vi "Serial_numberExt_429B.vi"(10 "PCBA Barcode":string="SVI77664916000894", 11 "Test Operator ID":string="13984") -> (0 "Check SUM HEX":string, 1 "Serial number (Hex)":string, 3 "ProgrammingResult":bool)   [LabVIEW 2018]
panel:
  out "concatenated string 2":string
  out "cmd1":string
  out "MUX RELAY":refnum<visa-resource-name>
  out "Byte1":string
  out "Byte2":string
  out "Byte3":string
  out "Byte4":string
  out "Sum":string
  in  "CSV path":path=path "D:/20161122/LNK01E-213300ALF/Serial_Log.csv"
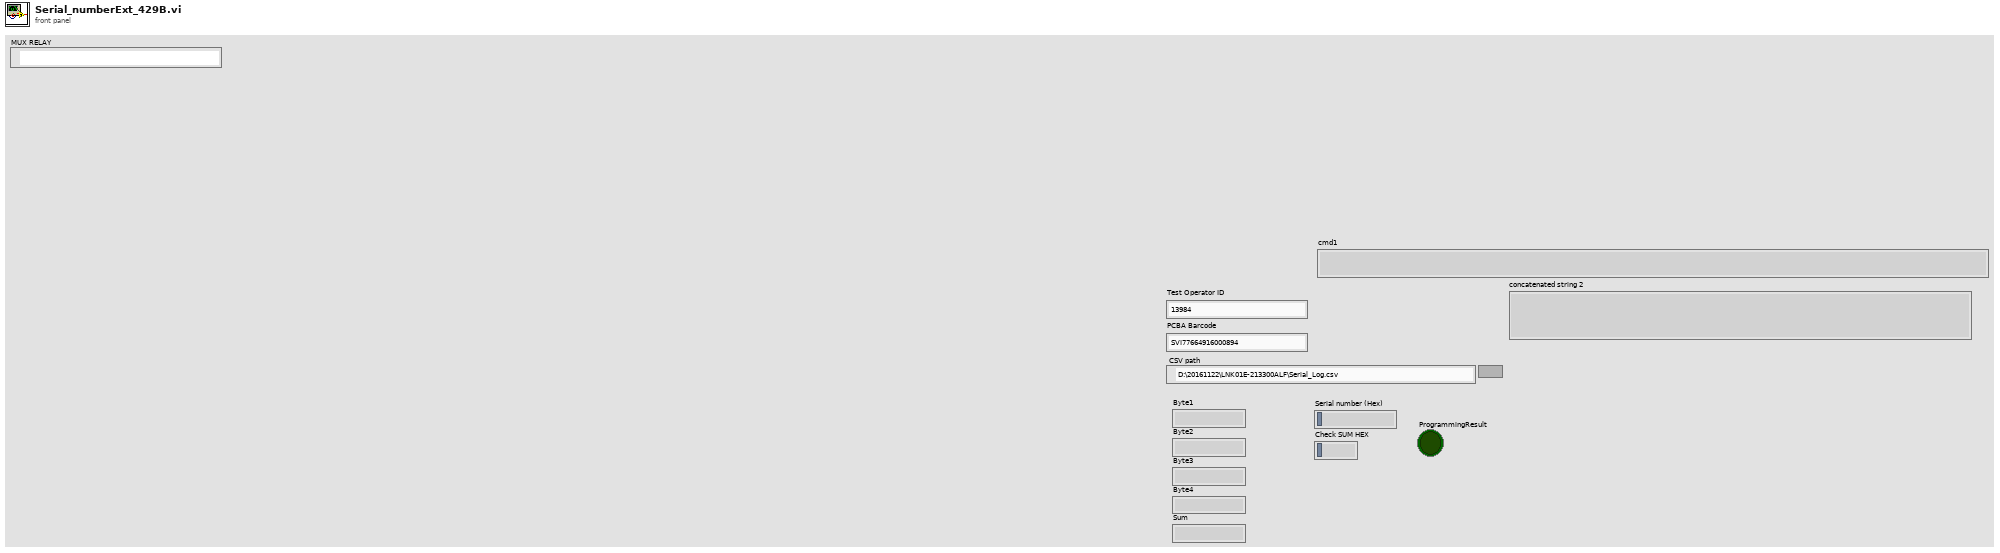
[diagram p1: front panel]
types:
  T1 = enum32{"Set Relay", "Append Relay", "Clear Relay", "Manual Cmd"}
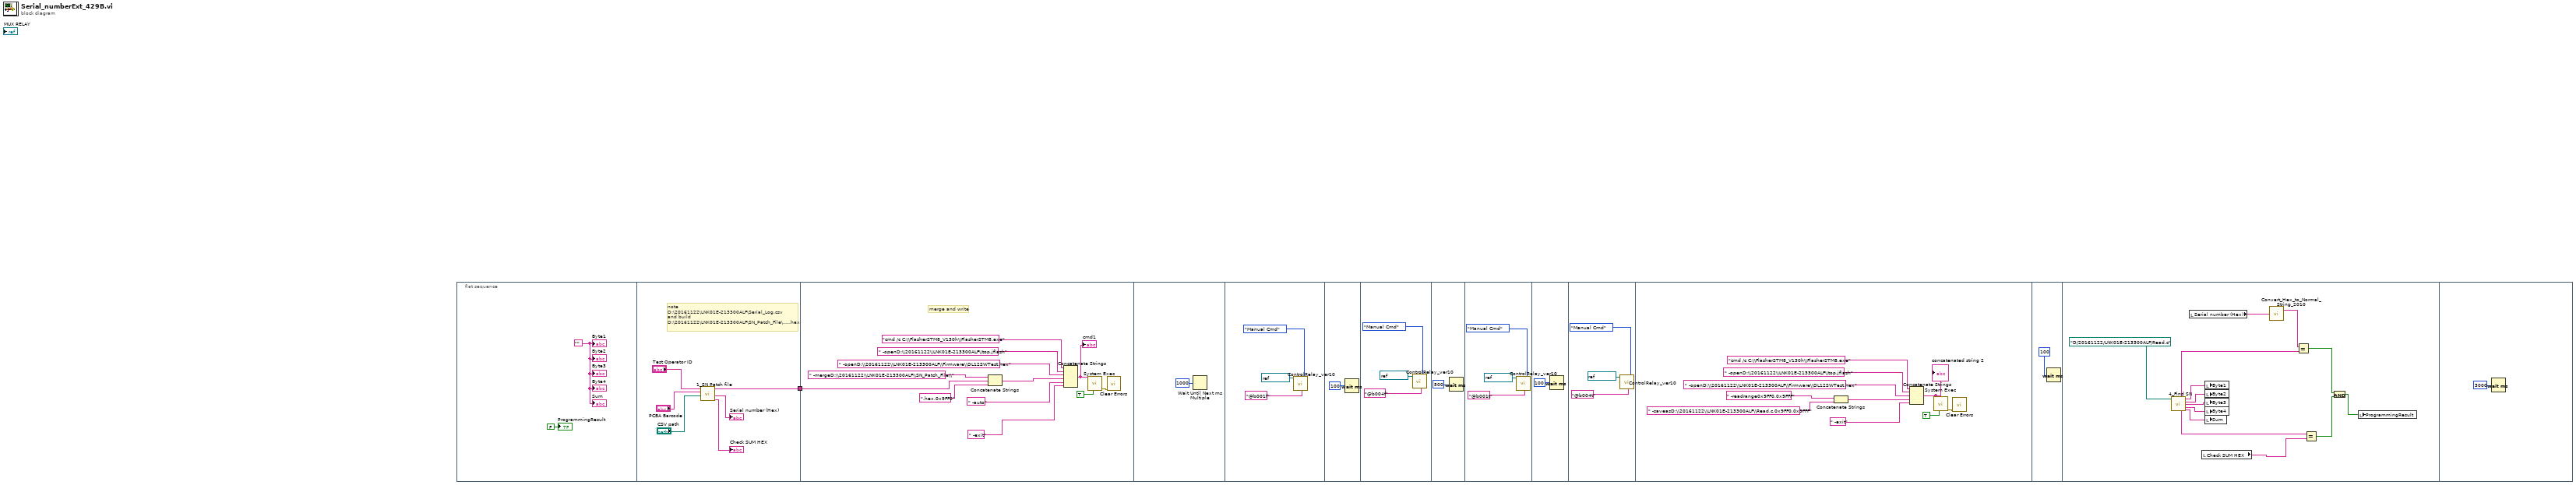
[diagram p0: block diagram]
diagram:
  n1 = flat-sequence {
    tunnel: [w6] -> w1
    tunnel: w1 -> [w14]
    frame #0 {
      w3 = ""
      "Sum" <- w3
      "Byte4" <- w3
      "Byte3" <- w3
      "Byte2" <- w3
      "Byte1" <- w3
      "ProgrammingResult" <- FALSE ("ProgrammingResult")
    }
    frame #1 {
      # "note\nD:\\20161122\\LNK01E-213300ALF\\Serial_Log.csv\nand build\nD:\\20161122\\LNK01E-213300ALF\\SN_Patch_File\\.....hex"
      n2 = call "1_SN Patch file.vi"("CSV path"="CSV path", "PCBA Barcode"="PCBA Barcode", "Test Operator ID"="Test Operator ID") -> ("Check SUM HEX"=→"Check SUM HEX":string, "Serial number (Hex)"=→"Serial number (Hex)":string, "PCBA Barcode out"=w6:string)  [unwired: 5 in, 1 out]
    }
    frame #2 {
      # "merge and write"
      n3 = Concatenate Strings(" -mergeD:\\20161122\\LNK01E-213300ALF\\SN_Patch_File\\" ("command line"), w14, ".hex,0x9FF0" ("command line")) -> (w15:string)
      n4 = Concatenate Strings("cmd /c C:\\FlasherSTM8_V130h\\FlasherSTM8.exe" ("command line"), " -openD:\\20161122\\LNK01E-213300ALF\\top.jflash" ("command line"), " -openD:\\20161122\\LNK01E-213300ALF\\Firmware\\DL12SWTest.hex" ("command line"), w15, " -auto" ("command line"), " -exit" ("command line")) -> (w18:string)
      "cmd1" <- w18
      n5 = call <vilib>:"System Exec.vi"("run minimized? (F)"=TRUE, "command line"=w18) -> ("error out"=w17:errorcluster)  [unwired: 6 in, 3 out]
      n6 = call <vilib>:"Clear Errors.vi"("error in (no error)"=w17) -> ()  [unwired: 5 in, 2 out]
    }
    frame #3 {
      n7 = Wait Until Next ms Multiple(millisecond multiple=u32 1000) -> ()  [unwired: 1 out]
    }
    frame #4 {
      n8 = call "ControlRelay_ver10.vi"("VISA session"=refnum<visa-resource-name> "COM1", "write buffer"="@b001f", "Relay Setting"=T1."Manual Cmd") -> ()  [unwired: 13 in, 4 out]
    }
    frame #5 {
      n9 = Wait (ms)(milliseconds to wait=u32 100 ("millisecond multiple")) -> ()  [unwired: 1 out]
    }
    frame #6 {
      n10 = call "ControlRelay_ver10.vi"("VISA session"=refnum<visa-resource-name> "COM1", "write buffer"="@b004f", "Relay Setting"=T1."Manual Cmd") -> ()  [unwired: 13 in, 4 out]
    }
    frame #7 {
      n11 = Wait (ms)(milliseconds to wait=u32 500 ("millisecond multiple")) -> ()  [unwired: 1 out]
    }
    frame #8 {
      n12 = call "ControlRelay_ver10.vi"("VISA session"=refnum<visa-resource-name> "COM1", "write buffer"="@b001t", "Relay Setting"=T1."Manual Cmd") -> ()  [unwired: 13 in, 4 out]
    }
    frame #9 {
      n13 = Wait (ms)(milliseconds to wait=u32 100 ("millisecond multiple")) -> ()  [unwired: 1 out]
    }
    frame #10 {
      n14 = call "ControlRelay_ver10.vi"("VISA session"=refnum<visa-resource-name> "COM1", "write buffer"="@b004t", "Relay Setting"=T1."Manual Cmd") -> ()  [unwired: 13 in, 4 out]
    }
    frame #11 {
      n15 = Concatenate Strings(" -readrange0x9FF0,0x9FFF" ("command line"), " -saveasD:\\20161122\\LNK01E-213300ALF\\Read.c,0x9FF0,0x9FFF" ("command line")) -> (w46:string)
      n16 = Concatenate Strings("cmd /c C:\\FlasherSTM8_V130h\\FlasherSTM8.exe" ("command line"), " -openD:\\20161122\\LNK01E-213300ALF\\top.jflash" ("command line"), " -openD:\\20161122\\LNK01E-213300ALF\\Firmware\\DL12SWTest.hex" ("command line"), w46, " -exit" ("command line")) -> (w43:string)
      "concatenated string 2" <- w43
      n17 = call <vilib>:"System Exec.vi"("run minimized? (F)"=TRUE, "command line"=w43) -> ("error out"=w44:errorcluster)  [unwired: 6 in, 3 out]
      n18 = call <vilib>:"Clear Errors.vi"("error in (no error)"=w44) -> ()  [unwired: 5 in, 2 out]
    }
    frame #12 {
      n19 = Wait (ms)(milliseconds to wait=u32 100) -> ()  [unwired: 1 out]
    }
    frame #13 {
      n20 = call "4_Find SN.vi"("file (use dialog)"=path "D:/20161122/LNK01E-213300ALF/Read.c") -> ("SN"=w54:string, "Byte1"=w61:string, "Byte2"=w60:string, "Byte3"=w59:string, "Byte4"=w58:string, "SUM"=w53:string, "Sum"=w57:string)  [unwired: 8 in]
      n21 = local read "Serial number (Hex)"() -> (w56:string)
      n22 = local read "Check SUM HEX"() -> (w50:string)
      n23 = local write "Byte1"(w61) -> ()
      n24 = local write "Byte2"(w60) -> ()
      n25 = local write "Byte3"(w59) -> ()
      n26 = local write "Byte4"(w58) -> ()
      n27 = local write "Sum"(w57) -> ()
      n28 = call "Convert_Hex_to_Normal_String_2010.vi"("Initial Hex String"=w56) -> ("Normal String - Number to Hexadecimal String Method"=w55:string)  [unwired: 1 out]
      n29 = Equal?(x=w55, y=w54) -> (x = y?=w52:bool)
      n30 = Equal?(x=w53, y=w50) -> (x = y?=w51:bool)
      n31 = And(x=w52, y=w51) -> (x .and. y?=w49:bool)
      n32 = local write "ProgrammingResult"(w49) -> ()
    }
    frame #14 {
      n33 = Wait (ms)(milliseconds to wait=u32 3000) -> ()  [unwired: 1 out]
    }
  }
